vi "Default Value State Name.vi"() -> (4 "Set Default Value State":string, 6 "Initialize State":string, 8 "Post UI Update":string, 10 "Load Values":string)   [LabVIEW 2021, in "Converter Reusables.lvlib"]
uses:
  Converter Reusables.lvlib
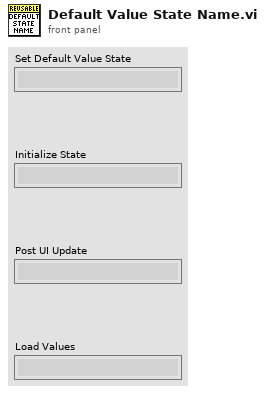
[diagram p1: front panel]
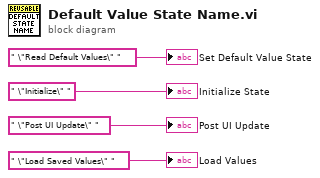
[diagram p0: block diagram]
diagram:
  "Set Default Value State" <- " \"Read Default Values\" " ("element")
  "Initialize State" <- " \"Initialize\" " ("new element/subarray")
  "Post UI Update" <- " \"Post UI Update\" " ("new element/subarray")
  "Load Values" <- " \"Load Saved Values\" " ("new element/subarray")
